vi "confirm button.vi"() -> (1 "T button?":bool)   [LabVIEW 2015, in "Biblioteka moduł map v3.lvlib" / "task erl.lvlib"]
uses:
  task erl.lvlib
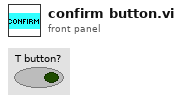
[diagram p1: front panel]
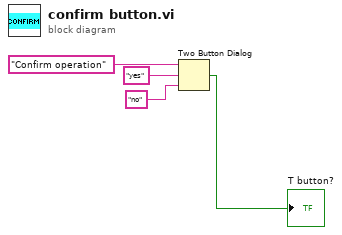
[diagram p0: block diagram]
diagram:
  n1 = Two Button Dialog(message="Confirm operation", 1:"no" ("F button name (\"Cancel\")"), 2:"yes" ("T button name (\"OK\")")) -> (T button?=→"T button?":bool)
